vi "Compare Axis Methods.vi"() -> ()   [LabVIEW 2014]
uses:
  Spectral Data.ctl
panel:
  in  "Saved":T1
  in  "Measured":T1
  out "Residues Raman Shift":cluster{i32[], "Raman Shift":dbl[]}(graph)
  out "Residues Energy":cluster{i32[], "Energy":dbl[]}(graph)
  out "Residues Wavelength":cluster{i32[], "Wavelength":dbl[]}(graph)
  # "LICENSED MATERIALS – PROPERTY OF IBM\nCopyright IBM Corp. 2016,\nALL RIGHTS RESERVED"
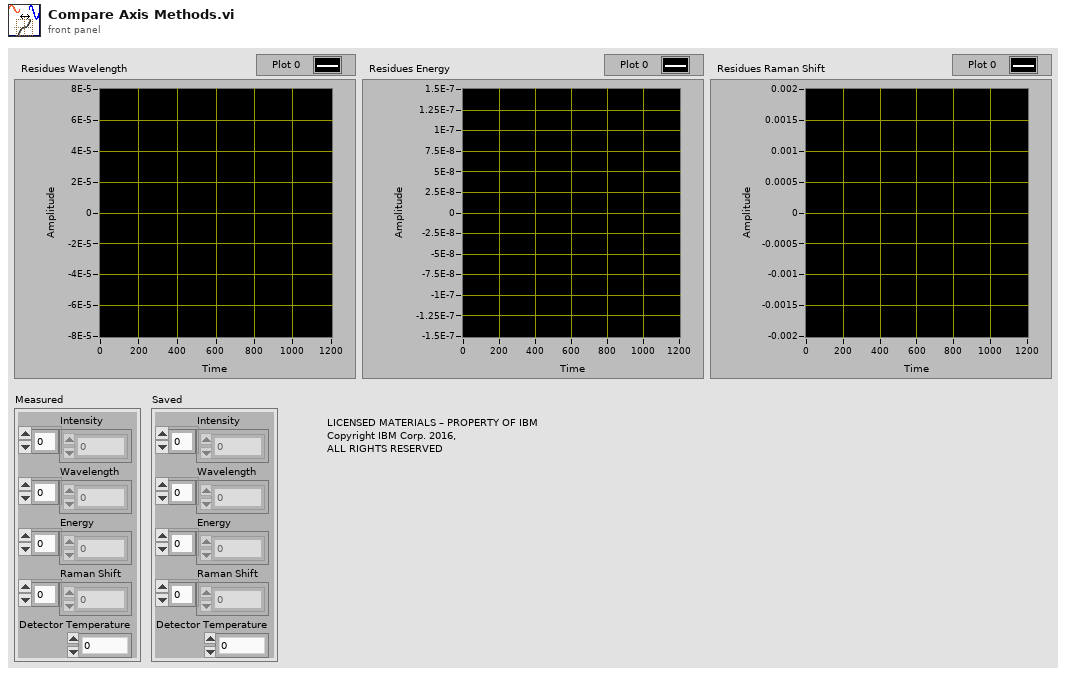
[diagram p1: front panel]
types:
  T1 = typedef "Spectral Data.ctl" = cluster{"Intensity":dbl[], "Wavelength":dbl[], "Energy":dbl[], "Raman Shift":dbl[], "Detector Temperature":dbl}
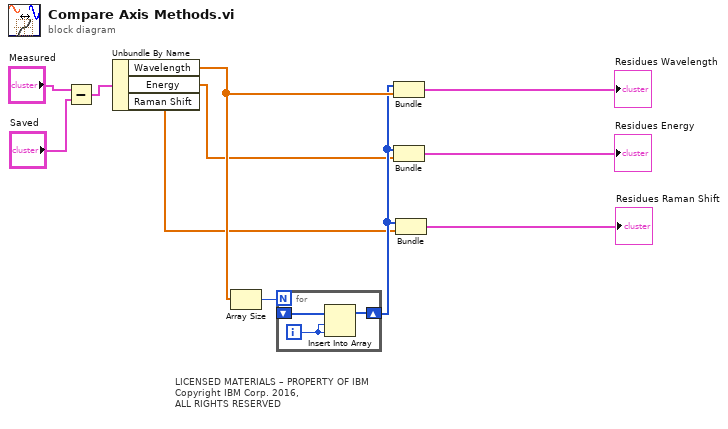
[diagram p0: block diagram]
diagram:
  # "LICENSED MATERIALS – PROPERTY OF IBM\nCopyright IBM Corp. 2016,\nALL RIGHTS RESERVED"
  n1 = Subtract(x="Measured", y="Saved") -> (x-y=w1:T1)
  n2 = Unbundle By Name(w1) -> ("Wavelength"=w11:dbl[], "Energy"=w8:dbl[], "Raman Shift"=w7:dbl[])
  n3 = Array Size(array=w11) -> (size(s)=w10:i32)
  n4 = for {
    N: w10 -> [_]
    shift-right: [w13] -> w9
    shift-left: _ -> [w12]
    i -> [w14]
    n5 = Insert Into Array(array=w12, index=w14, new element=w14) -> (w13:i32[])
  }
  n6 = Bundle(w9, "Wavelength"=w11) -> (→"Residues Wavelength":cluster{i32[], "Wavelength":dbl[]})  [unwired: 1 in]
  n7 = Bundle(w9, "Energy"=w8) -> (→"Residues Energy":cluster{i32[], "Energy":dbl[]})  [unwired: 1 in]
  n8 = Bundle(w9, "Raman Shift"=w7) -> (→"Residues Raman Shift":cluster{i32[], "Raman Shift":dbl[]})  [unwired: 1 in]
